vi "updateILCOutputs.vi"(8 "error in (no error)":errorcluster, 11 "Model in":refnum<class "Model.lvclass">) -> (0 "error out":errorcluster, 3 "Model out":refnum<class "Model.lvclass">)   [LabVIEW 2015, in "Model.lvclass"]
uses:
  Model.lvclass
  <userlib>/Common/ILC/Typedefs/OutputData.ctl
  Model.lvclass/Model.ctl
  <userlib>/Common/Devices/PressureValve/PressureValve/PressureValve.lvclass/PressureValve.ctl
  <userlib>/Common/ILC/ILC/ILC.lvclass/ILC.ctl
  <userlib>/Common/ILC/ILC/ILC.lvclass
  <userlib>/Common/ILC/Typedefs/ILCTypedefs.lvlib
  <userlib>/Common/Devices/PressureValve/PressureValve/PressureValve.lvclass
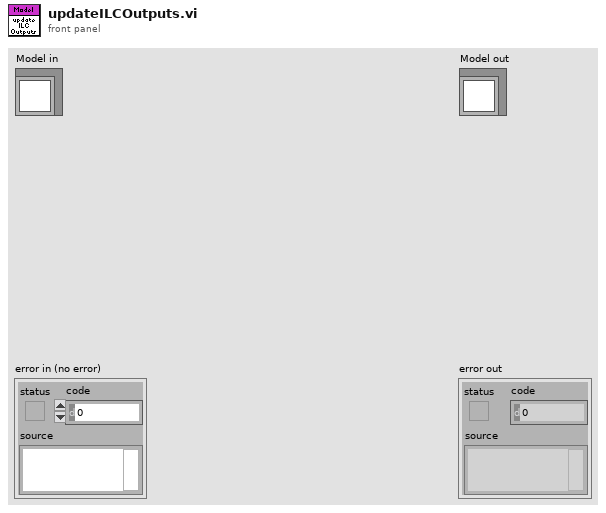
[diagram p1: front panel]
types:
  T1 = typedef "ILCCommon.lvlib/ILCTypedefs.lvlib/OutputData.ctl" = cluster{"Step & Direction":i16, "Blower RPM":u8, "PWM (SSR)":u8, "Ch1":u16, "Ch2":u16, "Ch3":u16, "Ch4":u16}
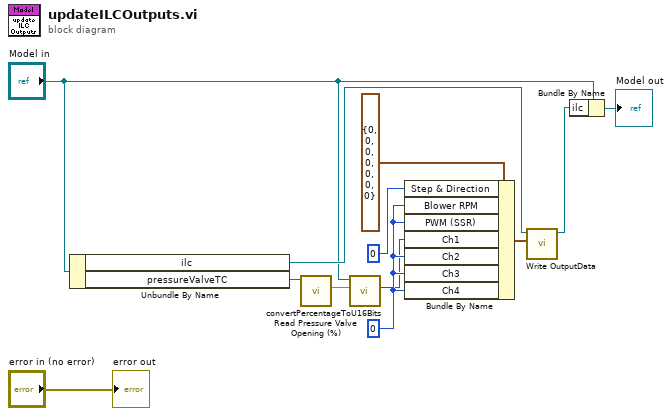
[diagram p0: block diagram]
diagram:
  w6 = u8 0 ("Blower RPM")
  n1 = Unbundle By Name("Model in") -> ("ilc"=w11:refnum<class "ILC.lvclass">, "pressureValveTC"=w5:refnum<class "PressureValveTC.lvclass">)
  n2 = call <userlib>:"Read Pressure Valve Opening (%).vi"("PressureValve in"=w5) -> ("Pressure Valve Opening (%)"=w1:dbl)  [unwired: 9 in, 1 out]
  n3 = call "convertPercentageToU16Bits.vi"("Percentage (%)"=w1, "Model in"="Model in") -> ("u16Equivalent"=w4:u16)  [unwired: 7 in, 2 out]
  n4 = Bundle By Name(cluster=T1 {"Step & Direction"=0, "Blower RPM"=0, "PWM (SSR)"=0, "Ch1"=0, "Ch2"=0, "Ch3"=0, "Ch4"=0} ("OutputData"), "Step & Direction"=i16 0, "Blower RPM"=w6, "PWM (SSR)"=w6, "Ch1"=w4, "Ch2"=w6, "Ch3"=w6, "Ch4"=w6) -> (w7:T1)
  n5 = call <userlib>:"Write OutputData.vi"("OutputData"=w7, "ILC in"=w11) -> ("ILC out"=w8:refnum<class "ILC.lvclass">)  [unwired: 9 in]
  n6 = Bundle By Name(cluster="Model in", "ilc"=w8) -> (→"Model out":refnum<class "Model.lvclass">)
  "error out" <- "error in (no error)"
